vi "out reselt.vi"(8 "error in":errorcluster, 9 "status":bool, 10 "serial":string, 11 "Module ID":i32=-1) -> (0 "error out":errorcluster)   [LabVIEW 2024, in "cameraV1.lvlib"]
doc: "_____\nCreated using DQMH Framework: Event Scripter 7.1.0.1503."
uses:
  cameraV1.lvlib
  out reselt Argument--cluster.ctl
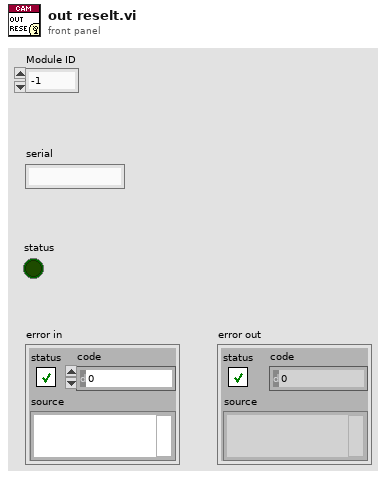
[diagram p1: front panel]
types:
  T1 = typedef "cameraV1.lvlib/out reselt Argument--cluster.ctl" = cluster{"Module ID":i32, "serial":string, "status":bool}
  T2 = typedef "cameraV1.lvlib/Broadcast Events--cluster.ctl" = cluster{"Module Did Init":refnum<user-event>, "Status Updated":refnum<user-event>, "Error Reported":refnum<user-event>, "Module Did Stop":refnum<user-event>, "Update Module Execution Status":refnum<user-event>, "out reselt":refnum<user-event>}
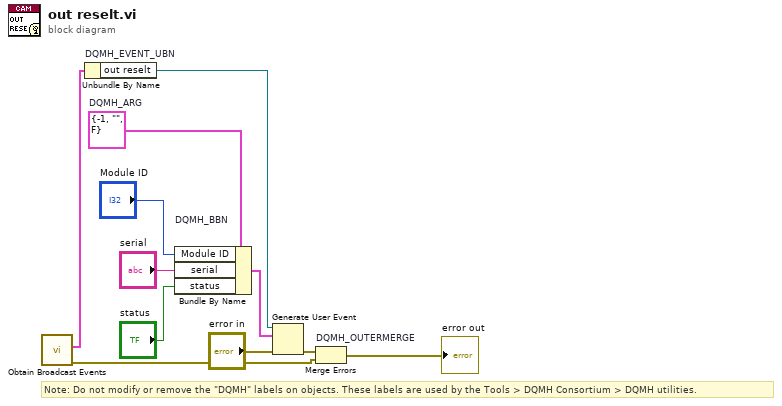
[diagram p0: block diagram]
diagram:
  w6 = T1 {"Module ID"=-1, "serial"="", "status"=FALSE}  # DQMH_ARG
  # "Note: Do not modify or remove the \"DQMH\" labels on objects. These labels are used by the Tools > DQMH Consortium > DQMH utilities."
  n1 = call "Obtain Broadcast Events.vi"() -> ("error out"=w2:errorcluster, "cameraV1 Broadcast Events"=w1:T2)  [unwired: 10 in]
  n2 = Unbundle By Name "DQMH_EVENT_UBN"(w1) -> ("out reselt"=w8:refnum<user-event>)
  n3 = Bundle By Name "DQMH_BBN"(cluster=w6, "Module ID"="Module ID", "serial"="serial", "status"="status") -> (w9:T1)
  n4 = Generate User Event(user event=w8, event data cluster=w9, error in="error in") -> (error out=w7:errorcluster)  [unwired: 1 in, 1 out]
  n5 = Merge Errors "DQMH_OUTERMERGE"(w7, w2) -> (→"error out":errorcluster)
